vi "Google Earth - Camera Position - Write.vi"(8 "error in":errorcluster, 9 "speed":dbl, 10 "Camera Position":T1={"Azimuth"=0.0, "FocusPointAltitude"=0.0, "FocusPointLatitude"=0.0, "FocusPointLongitude"=0.0, "Range"=0.0, "Tilt"=0.0, "altMode"=1} {"altMode" items=["RelativeToGroundAltitudeGE", "AbsoluteAltitudeGE"]}, 11 "Refnum in":refnum<k7>) -> (0 "error out":errorcluster, 3 "Refnum Out":refnum<k7>)   [LabVIEW 8.6]
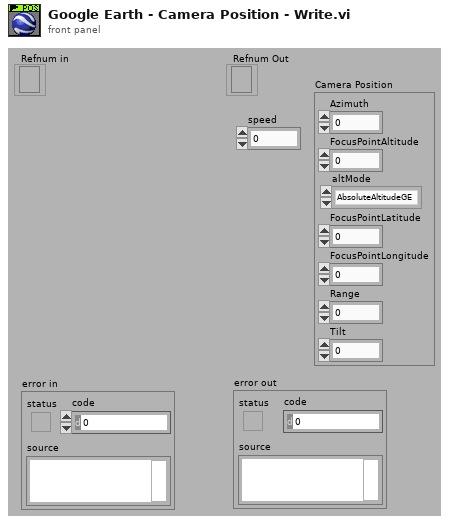
[diagram p1: front panel]
types:
  T1 = cluster{"Azimuth":dbl, "FocusPointAltitude":dbl, "FocusPointLatitude":dbl, "FocusPointLongitude":dbl, "Range":dbl, "Tilt":dbl, "altMode":i32}
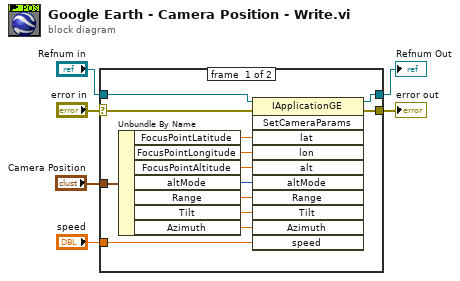
[diagram p0: block diagram]
diagram:
  n1 = case shown="No Error" "error in" {
    selector: "error in" -> [w7 w21]
    tunnel: [w19 w20] -> w6
    tunnel: "Refnum in" -> [w18 w20]
    tunnel: [w17 w21] -> w4
    tunnel: "speed" -> [w10 _]
    tunnel: "Camera Position" -> [w8 _]
    frame #0 {
      n2 = Unbundle By Name(w8) -> ("FocusPointLatitude"=w16:dbl, "FocusPointLongitude"=w15:dbl, "FocusPointAltitude"=w14:dbl, "altMode"=w9:i32, "Range"=w13:dbl, "Tilt"=w12:dbl, "Azimuth"=w11:dbl)
      n3 = invoke class="IApplicationGE" method="SetCameraParams"(reference=w18, error in=w7, "lat"=w16, "lon"=w15, "alt"=w14, "altMode"=w9, "Range"=w13, "Tilt"=w12, "Azimuth"=w11, "speed"=w10) -> (reference out=w19:refnum<k7>, error out=w17:errorcluster)  [unwired: 1 in, 9 out]
    }
    frame #1 {
    }
  }
  "error out" <- w4
  "Refnum Out" <- w6
